vi "CurrentInstance.vi"(11 "error in (no error)":errorcluster) -> (15 "error out":errorcluster)   [LabVIEW 2016, in "Drona Test.lvlib"]
uses:
  Drona Test.lvlib
  main/apis/Setup/GetVI/GetVIByPath.vi
  main/apis/Stimulus/VI/RunVI.vi
  main/apis/Stimulus/VI/MakeVIFrontMost.vi
  <vilib>/addons/_JKI Toolkits/Caraya/classes/Assert/Assert Not Error.vi
  main/Drona.lvlib
  main/apis/Setup/GetVI/GetVI.lvlib
  main/apis/Stimulus/VI/VI.lvlib
  <vilib>/addons/_JKI Toolkits/Caraya/classes/Assert/Assert.lvclass
  <vilib>/addons/_JKI Toolkits/Caraya/classes/Test/Test.lvclass
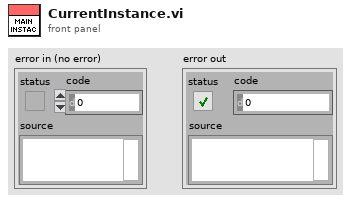
[diagram p1: front panel]
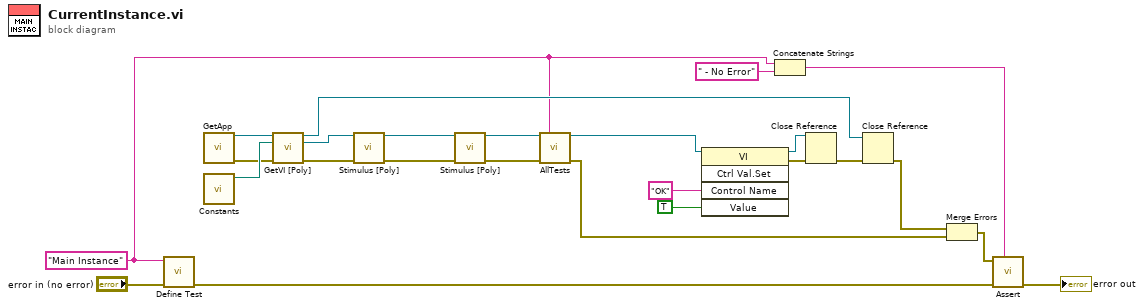
[diagram p0: block diagram]
diagram:
  w1 = "Main Instance" ("Label (VI Title)")
  n1 = call <vilib>:"Define Test.vi"("error in (no error)"="error in (no error)", "Label (VI Title)"=w1) -> ("error out"=w6:errorcluster)  [unwired: 9 in]
  n2 = call "GetApp.vi"() -> ("Application Ref"=w11:refnum<vi>, "error out"=w10:errorcluster)  [unwired: 14 in]
  n3 = call "Constants.vi"() -> ("HelperMain path"=w25:path)  [unwired: 9 in, 2 out]
  n4 = call-poly "GetVI [Poly].vi"("Application Ref in"=w11, "VI Path"=w25, "error in (no error)"=w10) -> ("Application Ref out"=w12:refnum<vi>, "VI Reference"=w13:refnum<vi>, "error out"=w14:errorcluster)  [unwired: 10 in]
  n5 = call-poly "Stimulus [Poly].vi"("VI Reference In"=w13, "error in"=w14) -> ("VI Reference Out"=w18:refnum<vi>, "error out"=w19:errorcluster)  [unwired: 12 in]
  n6 = call-poly "Stimulus [Poly].vi"("VI Reference In"=w18, "error in"=w19) -> ("VI Reference Out"=w16:refnum<vi>, "error out"=w15:errorcluster)  [unwired: 12 in]
  n7 = call "AllTests.vi"("VI in"=w16, "Label"=w1, "error in (no error)"=w15) -> ("VI out"=w17:refnum<vi>, "error out"=w4:errorcluster)  [unwired: 11 in]
  n8 = invoke class="VI" method="Ctrl Val.Set"(reference=w17, "Control Name"="OK", "Value"=TRUE) -> (reference out=w23:refnum<vi>, error out=w24:errorcluster)  [unwired: 2 in, 3 out]
  n9 = Concatenate Strings(w1, " - No Error" ("Label (VI Title)")) -> (w2:string)
  n10 = Close Reference(reference=w23, error in (no error)=w24) -> (error out=w20:errorcluster)
  n11 = Close Reference(reference=w12, error in (no error)=w20) -> (error out=w5:errorcluster)
  n12 = Merge Errors(w5, w4) -> (w9:errorcluster)
  n13 = call-poly <vilib>:"Assert.vi"("Label"=w2, "error in (no error)"=w6, "Not Error?"=w9) -> ("error out"=→"error out":errorcluster)  [unwired: 8 in]
